vi "RT Read Text File.vi"() -> ()   [LabVIEW 2018]
panel:
  in  "stop":bool
  in  "Boolean":bool
  out "text":string
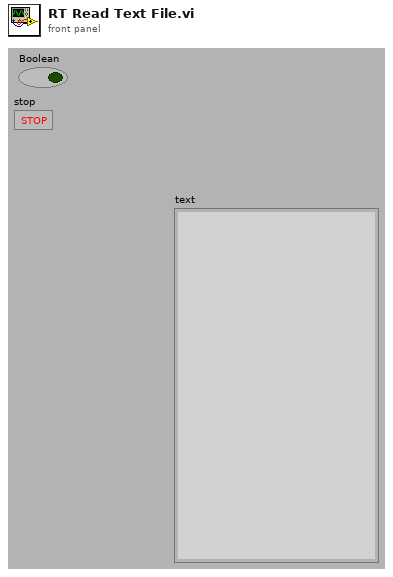
[diagram p1: front panel]
types:
  T1 = enum16{"open", "replace", "create", "open or create", "replace or create", "replace or create with confirmation"}
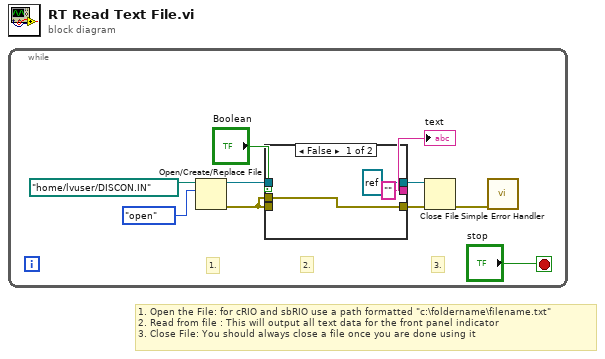
[diagram p0: block diagram]
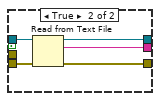
[diagram p2: hidden frame]
diagram:
  # "1. Open the File: for cRIO and sbRIO use a path formatted \"c:\\foldername\\filename.txt\"\n2. Read from file : This will output all text data for the front panel indicator\n3. Close File: You should always close a file once you are done using it"
  n1 = while {
    stop <- "stop" stop-if-true
    # "3."
    # "2."
    # "1."
    n2 = Open/Create/Replace File(file path (use dialog)=path "/home/lvuser/DISCON.IN", operation (0:open)=T1."open") -> (refnum out=w4:refnum<file>, error out=w2:errorcluster)  [unwired: 4 in, 1 out]
    n3 = case shown="False" "Boolean" {
      tunnel: ["" w18] -> w10
      tunnel: [w12 w17] -> w9
      tunnel: [refnum<file> refnum ("refnum out") w16] -> w8
      tunnel: w4 -> [_ w15]
      tunnel: w2 -> [_ w14]
      tunnel: w2 -> [w12 _]
      frame False {
      }
      frame True {
        n4 = Read from Text File(file (use dialog)=w15, error in=w14) -> (refnum out=w16:refnum<file>, text=w18:string, error out=w17:errorcluster)  [unwired: 2 in, 1 out]
      }
    }
    "text" <- w10
    n5 = Close File(refnum=w8, error in=w9) -> (error out=w7:errorcluster)  [unwired: 1 out]
    n6 = call <vilib>:"Simple Error Handler.vi"("error in (no error)"=w7) -> ()  [unwired: 4 in, 5 out]
  }
